vi "VisionTest3.vi"() -> ()   [LabVIEW 2011]
panel:
  out "Ready":bool
  in  "Take Pics":bool
  out "Processed Image 2":T1(plugin-control)
  out "Processed Image 1":T1(plugin-control)
  out "Original Image 2":T1(plugin-control)
  out "Original Image 1":T1(plugin-control)
  out "Final Image":T1(plugin-control)
  out "Dist Error":dbl
  out "Vertical Angle Error":dbl
  out "Target Dist":dbl
  out "Vertical Angle":dbl
  out "Horizontal Angle":dbl
  in  "Green Range":cluster{"Lower value":i32, "Upper value":i32}={"Lower value"=0, "Upper value"=255}
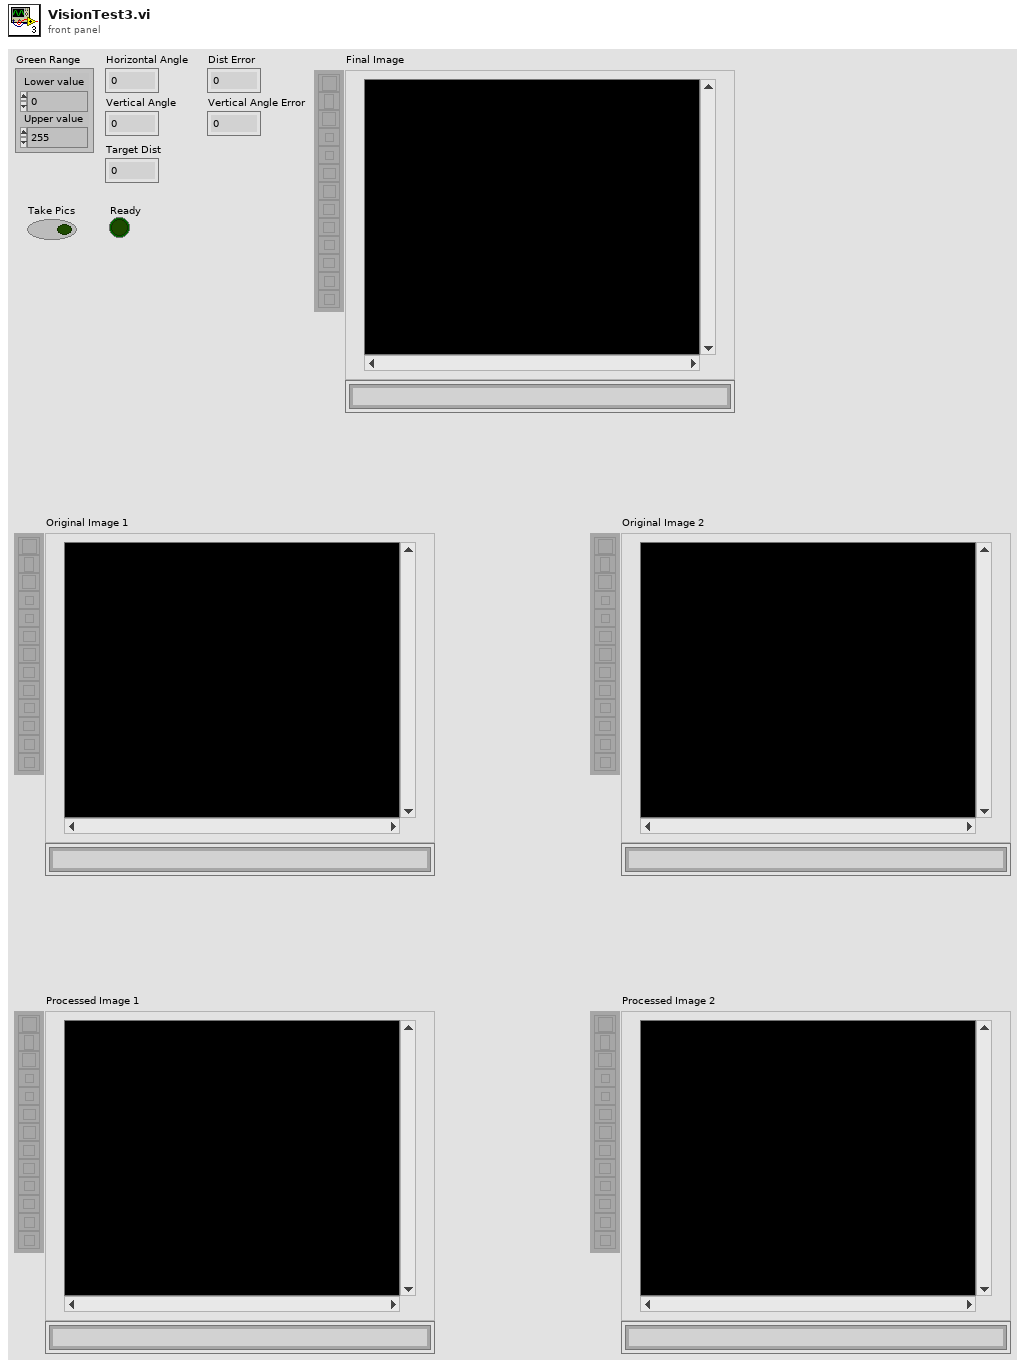
[diagram p1: front panel]
types:
  T1 = typedef "IMAQ Image.ctl" = refnum<image>
  T2 = typedef "WPI_CameraDevRef.ctl" = cluster{"Camera Address":string, "CameraStatus":errorcluster, "Acquire Image Notifier":refnum<notifier>}
  T3 = cluster{"Image 1":T1, "Image 2":T1, "Rotated 1":T1, "Rotated 2":T1, "Processed 1":T1, "Processed 2":T1, "XOR Image":T1, "[7]":T1, "[8]":T1}
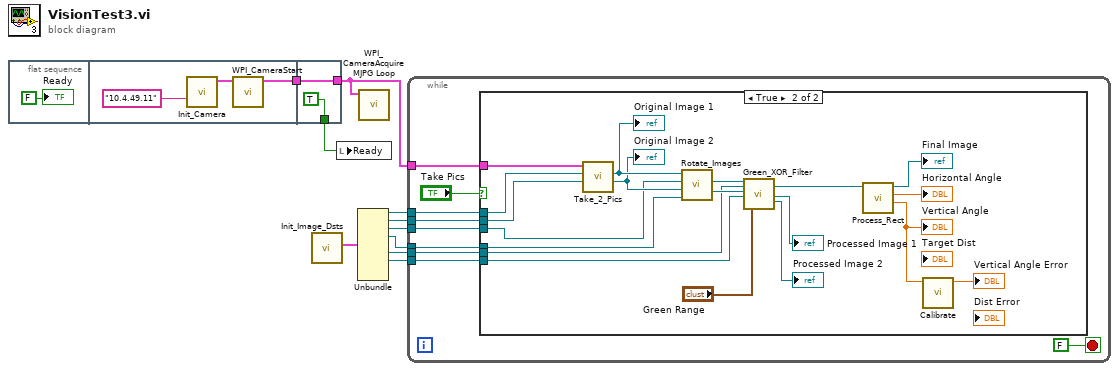
[diagram p0: block diagram]
diagram:
  n1 = flat-sequence {
    tunnel: [w14] -> w3
    tunnel: [w16] -> w1
    tunnel: w3 -> [w16]
    tunnel: [TRUE] -> w2
    frame #0 {
      "Ready" <- FALSE
    }
    frame #1 {
      n2 = call "Init_Camera.vi"("Camera IP"="10.4.49.11") -> ("CameraDevRef Out"=w12:T2)  [unwired: 10 in]
      n3 = call <vilib>:"WPI_CameraStart.vi"("CameraDevRef"=w12) -> ("CameraDevRef Out"=w14:T2)  [unwired: 9 in, 1 out]
    }
    frame #2 {
    }
  }
  n4 = call "Init_Image_Dsts.vi"() -> ("Image Dsts Out"=w10:T3)  [unwired: 11 in]
  n5 = local write "Ready"(w2) -> ()
  n6 = Unbundle(w10) -> ("Image 1"=w9:T1, "Image 2"=w8:T1, "Rotated 1"=w7:T1, "Rotated 2"=w6:T1, "Processed 2"=w5:T1, "XOR Image"=w4:T1)  [unwired: 3 out]
  n7 = call <vilib>:"WPI_CameraAcquire MJPG Loop.vi"("CameraDevRef"=w1) -> ()  [unwired: 11 in]
  n8 = while {
    tunnel: w1 -> [w25]
    tunnel: w9 -> [w24]
    tunnel: w8 -> [w23]
    tunnel: w7 -> [w22]
    tunnel: w6 -> [w21]
    tunnel: w5 -> [w20]
    tunnel: w4 -> [w19]
    stop <- FALSE stop-if-true
    n9 = case shown="True" "Take Pics" {
      tunnel: w25 -> [_ w34]
      tunnel: w24 -> [_ w31]
      tunnel: w23 -> [_ w30]
      tunnel: w22 -> [_ w29]
      tunnel: w21 -> [_ w28]
      tunnel: w20 -> [_ w27]
      tunnel: w19 -> [_ w26]
      frame False {
      }
      frame True {
        n10 = call "Take_2_Pics.vi"("Image Src Dark"=w30, "Image Src Light"=w31, "CameraDevRef"=w34) -> ("Image Out Dark"=w35:T1, "Image Out Light"=w36:T1)  [unwired: 7 in]
        "Original Image 1" <- w36
        "Original Image 2" <- w35
        n11 = call "Rotate_Images.vi"("Rotated Dst 2"=w28, "Image Src 2"=w35, "Rotated Dst 1"=w29, "Image Src 1"=w36) -> ("Rotated Image 2"=w37:T1, "Rotated Image 1"=w38:T1)  [unwired: 6 in]
        n12 = call "Green_XOR_Filter.vi"("Image Src 1"=w38, "Processed 1 Dst"=w27, "Image Src 2"=w37, "Processed 2 Dst"=w26, "Green Range"="Green Range") -> ("XOR Image"=w43:T1, "Processed Image 1"=→"Processed Image 1":T1, "Processed Image 2"=→"Processed Image 2":T1)  [unwired: 12 in]
        n13 = call "Process_Rect.vi"("Difference image"=w43) -> ("Vertical Angle"=w41:dbl, "Horizontal Angle"=→"Horizontal Angle":dbl, "Processed Image Out"=→"Final Image":T1)  [unwired: 5 in, 3 out]
        "Vertical Angle" <- w41
        n14 = call "Calibrate.vi"("Calculated Vertical Angle"=w41) -> ("Vertical Angle Error"=→"Vertical Angle Error":dbl)  [unwired: 10 in]
      }
    }
  }
